vi "RT Main.vi"() -> ()   [LabVIEW 2021]
uses:
  Real-Time/Controls/Data FGV Action.ctl
  Program Files (x86)/National Instruments/LabVIEW 2021/ProjectTemplates/Source/myRIO/Oscilloscope/myRIO v1.1/Real-Time/Controls/Wave Parameters.ctl
  Program Files (x86)/National Instruments/LabVIEW 2021/ProjectTemplates/Source/myRIO/Oscilloscope/myRIO v1.1/Real-Time/Controls/Waveform Enum.ctl
  Program Files (x86)/National Instruments/LabVIEW 2021/ProjectTemplates/Source/myRIO/Oscilloscope/myRIO v1.1/Real-Time/Controls/Channel Selector.ctl
  <vilib>/Platform/TimedLoop/XDataNode/timing_clust.ctl
  <vilib>/Platform/TimedLoop/XDataNode/nitl_modes.ctl
  <vilib>/Platform/TimedLoop/XDataNode/wakeup.ctl
  Real-Time/Controls/Global Stop.vi
  <vilib>/FPGAPlugInAG/myRIO-1900/niLvFpga_Open_myRIO-1900.vi
  <vilib>/rvi/interface/common/dynamic/niFpgaDynamicAddResources.vi
  <vilib>/rvi/interface/common/niFpgaWaitOnOcc.vi
  <vilib>/Utility/error.llb/Error Cluster From Error Code.vi
  <vilib>/rvi/errors/niLvFpgaAdjustHostInterfaceError.vi
  <vilib>/myRIO/Common/Instrument Driver Framework/Utilities/vis/FPGA Ref Manager.vi
  <vilib>/myRIO/Common/Instrument Driver Framework/Utilities/vis/Ref Counter.vi
  <vilib>/FPGAPlugInAG/Dynamic/niLvFpga_Run_Dynamic.vi
  <vilib>/rvi/Analysis/host/Private/Sample Rate To Loop Time (ticks).vi
  <vilib>/FPGAPlugInAG/Dynamic/niLvFpga_Abort_Dynamic.vi
  <vilib>/FPGAPlugInAG/Dynamic/niLvFpga_Close_Dynamic.vi
  <vilib>/rvi/interface/nirviOpenFPGA/nirviOpenFPGA.xnode
  FPGA Bitfiles/ScopeBitFile2CH.lvbitx
  <vilib>/rvi/interface/nirviMethod/nirviMethod.xnode
  <vilib>/rvi/interface/nirviReadWriteControl/nirviReadWriteControl.xnode
  <vilib>/Platform/TimedLoop/XDataNode/XDataNode.xnode
  <vilib>/rvi/interface/nirviCloseFPGA/nirviCloseFPGA.xnode
  <vilib>/rvi/errors/niLvFpgaMergeErrorWithErrorCode.vi
  <vilib>/rvi/interface/Simulation/niFpgaSimulationCallBeginRW.vi
  <vilib>/myRIO/Instrument Drivers/Utilities/Utilities.lvlib
  <vilib>/Platform/TimedLoop/XDataNode/XDNodeRunTimeDep.lvlib
  <vilib>/rvi/Analysis/host/Public/NI_FpgaMspHost.lvlib
  <vilib>/FPGAPlugInAG/Dynamic/niLvFpga_ConfigureFifo_Dynamic.vi
  <vilib>/FPGAPlugInAG/Dynamic/niLvFpga_StartFifo_Dynamic.vi
  NiFpgaLv.dll
  <vilib>/FPGAPlugInAG/Dynamic/niLvFpga_ReadFifo_Dynamic.vi
panel:
  in  "Number of Elements":u32=1000
  out "Elements Remaining":u32
  out "error out":errorcluster
  in  "Stop":bool
  out "End?":bool
  # "Instructions\n1. Run RT Main.vi\n2. Open Desktop Main.vi\n3. Specify myRIO IP Address\n4. Run Desktop Main.vi"
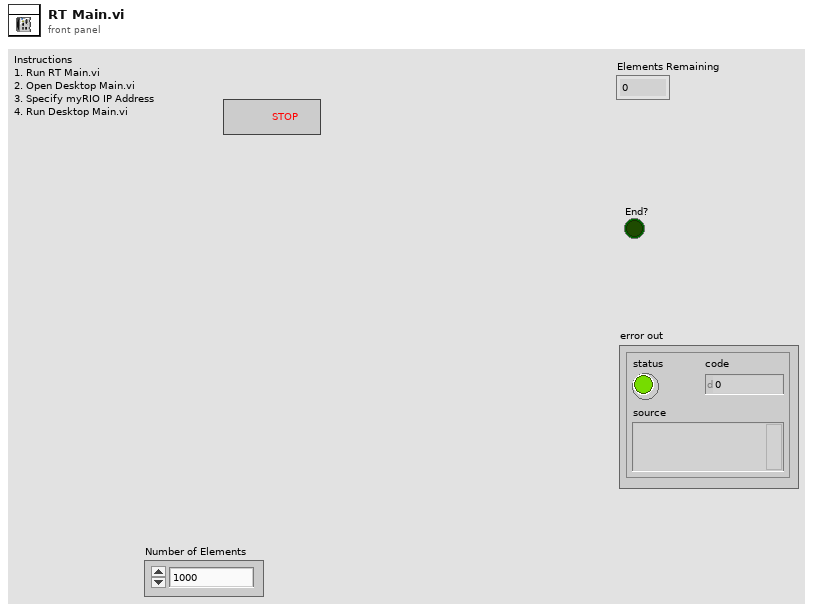
[diagram p1: front panel]
types:
  T1 = typedef "Data FGV Action.ctl" = enum16{"Initialize", "Set Scope Data", "Read Scope Data", "Set FGen", "Read FGen", "Set Params"}
  T2 = cluster{"read mode":enum16{"polling", "blocking"}, "write mode":enum16{"polling", "blocking"}}
  T3 = typedef "Wave Parameters.ctl" = cluster{"Frequency (Hz)":dbl, "Phase offset (deg)":dbl, "Vpeak (V)":dbl, "Offset (V)":dbl, "Waveform":T4, "Channel":T5}
  T4 = typedef "Waveform Enum.ctl" = enum16{"Sine", "Square"}
  T5 = typedef "Channel Selector.ctl" = enum16{"CH0", "CH1"}
  T6 = typedef "XDNodeRunTimeDep.lvlib/timing_clust.ctl" = cluster{"Expected End [f-1]":u64, "Actual End [f-1]":u64, "Finished Late? [f-1]":bool, "Expected End [i-1]":u64, "Actual End [i-1]":u64, "Finished Late? [i-1]":bool, "Expected Start [i]":u64, "Actual Start [i]":u64, "Expected Start [f]":u64, "Actual Start [f]":u64, "Source Name":string, "Structure Name":string, "Period":i64, "Deadline":i64, "Offset":i64, "Start":i64, "Priority":i32, "Timeout":i32, "Mode":T7, "Wakeup Reason":T8, "Error":errorcluster, "Source Type":string, "Secondary Source Type":string, "Global End Time":u64, "Global Start Time":u64, "Frame Duration":u64, "Iteration Duration":u64, "Assigned CPU":i32, "I/O Scan Engine Mode":u32}
  T7 = typedef "XDNodeRunTimeDep.lvlib/nitl_modes.ctl" = enum32{"No Change", "Process missed periods, maintain original phase", "Discard missed periods, maintain original phase", "Process missed periods, ignore original phase", "Discard missed periods, ignore original phase"}
  T8 = typedef "XDNodeRunTimeDep.lvlib/wakeup.ctl" = enum32{"Normal", "Aborted", "Asynchronous wakeup", "Timing source error", "Timed loop error", "Timeout"}
  T9 = typedef "Time Selector.ctl" = cluster{"Time/Div":T10}
  T10 = typedef "Time Knob.ctl" = dbl
  T11 = cluster{"Frequency (Hz)":bool, "Phase offset (deg)":bool, "Vpeak (V)":bool, "Offset (V)":bool, "Waveform":bool, "Channel":bool}
  T12 = typedef "Wave Properties - FPGA.ctl" = cluster{"Frequency (periods/tick)":fxp<+,32,0>, "Phase offset (periods)":fxp<+,32,0>, "Scale factor":fxp<+/-,24,1>, "Amplitude offset":fxp<+/-,24,12>, "Waveform":T4, "Channel":T5}
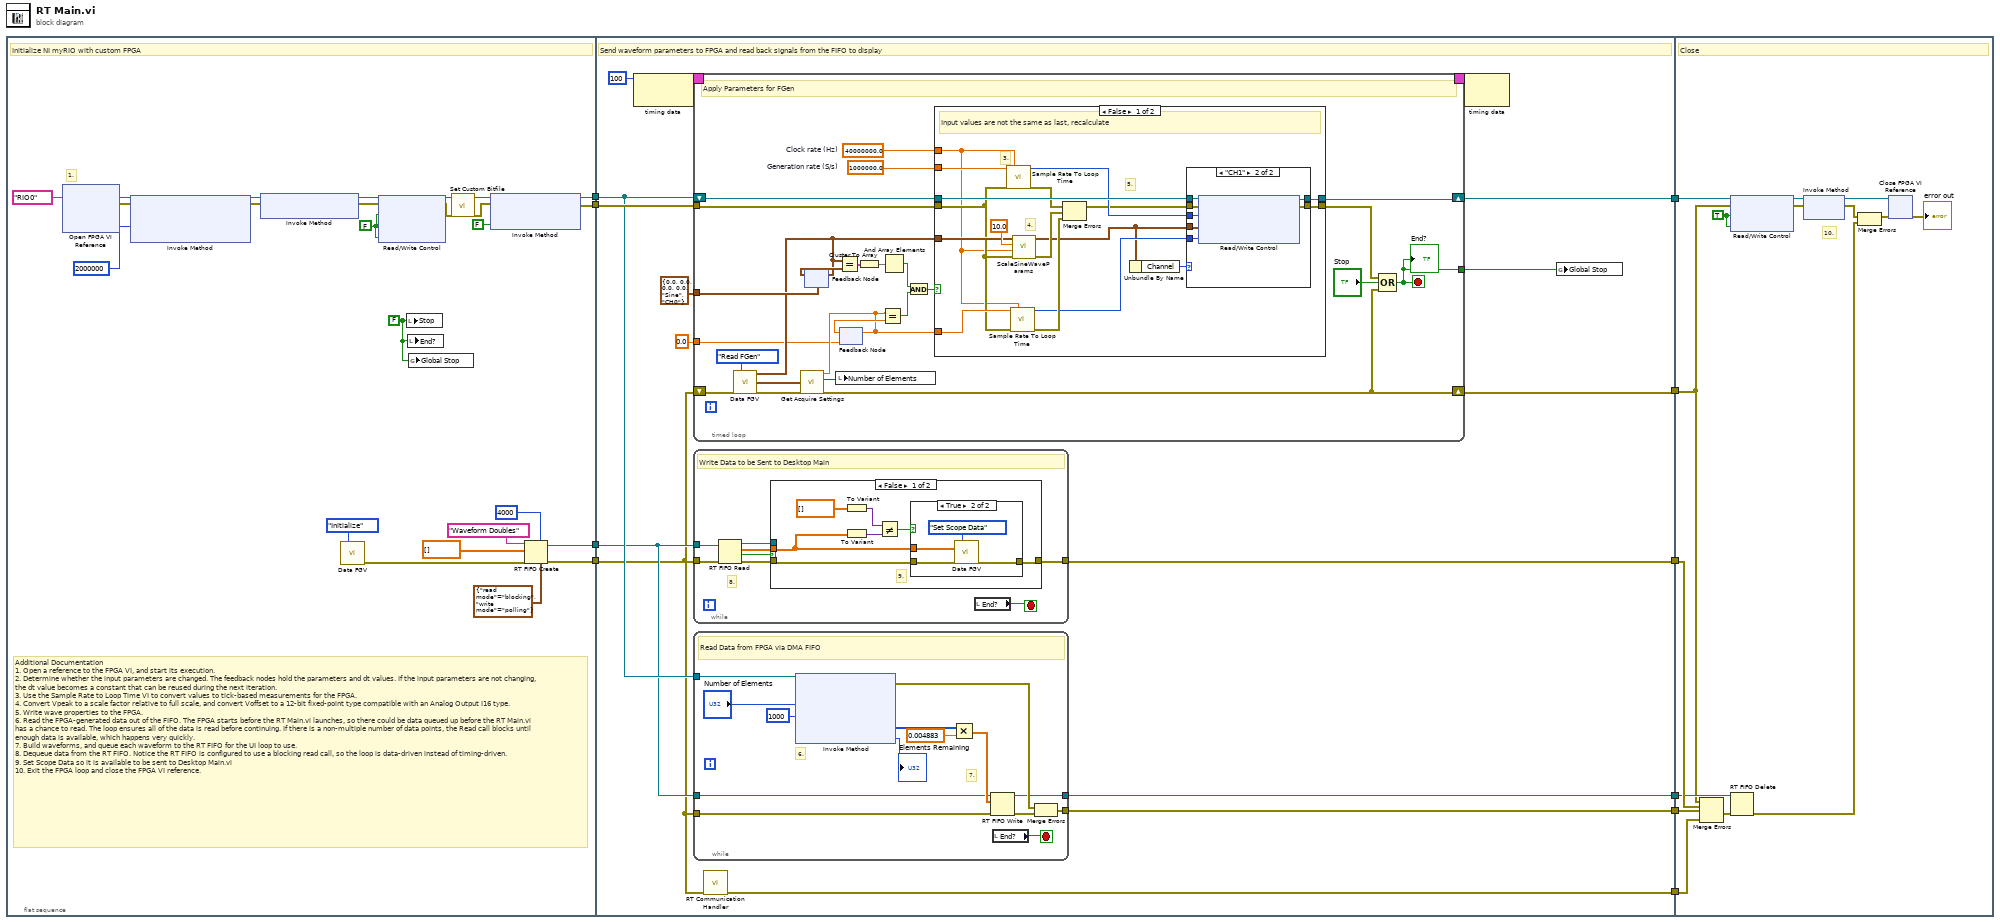
[diagram p0: block diagram]
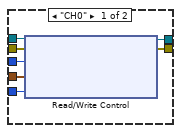
[diagram p4: hidden frame]
diagram:
  n1 = flat-sequence {
    tunnel: [w23] -> w10
    tunnel: [w22] -> w9
    tunnel: [w18] -> w6
    tunnel: [w17] -> w5
    tunnel: w10 -> [w44]
    tunnel: w9 -> [w51]
    tunnel: [w50] -> w8
    tunnel: [w45] -> w7
    tunnel: w6 -> [w37]
    tunnel: w5 -> [w42]
    tunnel: [w41] -> w4
    tunnel: [w40] -> w3
    tunnel: [w39] -> w2
    tunnel: [w36] -> w1
    tunnel: w8 -> [w165]
    tunnel: w7 -> [w151]
    tunnel: w4 -> [w158]
    tunnel: w3 -> [w157]
    tunnel: w2 -> [w156]
    tunnel: w1 -> [w152]
    frame #0 {
      w14 = FALSE ("Reset")
      w11 = FALSE ("Stop")
      # "Additional Documentation\n1. Open a reference to the FPGA VI, and start its execution.\n2. Determine whether the input parameters are changed. The feedback nodes hold the parameters and dt values. If the input parameters are not changing, the dt value becomes a constant that can be reused during the next iteration.\n3. Use the Sample Rate to Loop Time VI to convert values to tick-based measurements for the FPGA.\n4. Convert Vpeak to a scale factor relative to full scale, and convert Voffset to a 12-bit fixed-point type compatible with an Analog Output I16 type.\n5. Write wave properties to the FPGA. \n6. Read the FPGA-generated data out of the FIFO. The FPGA starts before the RT Main.vi launches, so there could be data queued up before the RT Main.vi has a chance to read. The loop ensures all of the data is read before continuing. If there is a non-multiple number of data points, the Read call blocks until enough data is available, which happens very quickly.\n7. Build waveforms, and queue each waveform to the RT FIFO for the UI loop to use.\n8. Dequeue data from the RT FIFO. Notice the RT FIFO is configured to use a blocking read call, so the loop is data-driven instead of timing-driven.\n9. Set Scope Data so it is available to be sent to Desktop Main.vi\n10. Exit the FPGA loop and close the FPGA VI reference."
      # "1."
      # "Initialize NI myRIO with custom FPGA"
      n2 = xnode "Open FPGA VI Reference"("resource name"=tag "RIO0") -> ("FPGA VI Reference Out"=w28:refnum<k20>, "error out"=w27:errorcluster)  [unwired: 1 in]
      n3 = xnode "Invoke Method"("FPGA VI Reference In"=w28, "error in"=w27, "Requested Depth"=u32 2000000) -> ("FPGA VI Reference Out"=w33:refnum<k20>, "error out"=w32:errorcluster)  [unwired: 1 out]
      n4 = xnode "Invoke Method"("FPGA VI Reference In"=w33, "error in"=w32) -> ("FPGA VI Reference Out"=w31:refnum<k20>, "error out"=w30:errorcluster)
      n5 = call "Data FGV.vi"("Action"=Data_FGV_Action."Initialize") -> ("error out"=w12:errorcluster)  [unwired: 10 in, 4 out]
      n6 = xnode "Read/Write Control"("FPGA VI Reference In"=w31, "error in"=w30, "Stop Output"=w11, "Initialize AO0"=w11, "Initialize AO1"=w11) -> ("FPGA VI Reference Out"=w29:refnum<k20>, "error out"=w26:errorcluster)
      n7 = local write "Stop"(w14) -> ()
      n8 = local write "End?"(w14) -> ()
      n9 = global write "Global Stop.vi" "Global Stop"(w14) -> ()
      n10 = call <vilib>:"Set Custom Bitfile.vi"("error in (no error)"=w26, "Custom FPGA Reference In"=w29) -> ("error out"=w24:errorcluster, "Custom FPGA Reference Out"=w25:refnum<k20>)  [unwired: 8 in]
      n11 = xnode "Invoke Method"("FPGA VI Reference In"=w25, "error in"=w24, "Wait Until Done (F)"=FALSE) -> ("FPGA VI Reference Out"=w23:refnum<k20>, "error out"=w22:errorcluster)
      n12 = RT FIFO Create(0:"Waveform Doubles" ("name (unnamed)"), 1:dbl[] [] ("x"), 3:w12, 6:u32 4000 ("size (10)"), 7:T2 {"read mode"=enum."blocking", "write mode"=enum."polling"} ("r/w modes (polling,polling)")) -> (8:w17:refnum<k33>, 11:w18:errorcluster)  [unwired: 3 in, 1 out]
    }
    frame #1 {
      # "Send waveform parameters to FPGA and read back signals from the FIFO to display"
      n13 = node-c288(i64 100 ("Period")) -> (w49:T6)
      n14 = while {
        tunnel: w42 -> [w72]
        tunnel: w37 -> [w67]
        tunnel: [w66] -> w40
        stop <- w73 stop-if-true
        # "8."
        # "Write Data to be Sent to Desktop Main"
        n15 = RT FIFO Read(0:w72, 3:w67) -> (8:w71:refnum<k33>, 9:w69:dbl[], 10:w68:bool, 11:w70:errorcluster)  [unwired: 2 in, 1 out]
        n16 = case shown="False" w68 {
          tunnel: w71 -> [_ _]
          tunnel: w70 -> [w75 w86]
          tunnel: w69 -> [w76 _]
          tunnel: [w74 w86] -> w66
          frame False {
            # "9."
            n17 = To Variant(anything=dbl[] [] ("x")) -> (Variant=w79:variant)
            n18 = To Variant(anything=w76) -> (Variant=w78:variant)
            n19 = Not Equal?(x=w79, y=w78) -> (x != y?=w77:bool)
            n20 = case shown="True" w77 {
              tunnel: w76 -> [_ w83]
              tunnel: w75 -> [w81 w85]
              tunnel: [w81 w82] -> w74
              frame False {
              }
              frame True {
                n21 = call "Data FGV.vi"("Action"=Data_FGV_Action."Set Scope Data", "Data"=w83, "error in (no error)"=w85) -> ("error out"=w82:errorcluster)  [unwired: 8 in, 4 out]
              }
            }
          }
          frame True {
          }
        }
        n22 = local read "End?"() -> (w73:bool)
      }
      n23 = timed-loop {
        shift-right: [w90] -> w50
        shift-left: w44 -> [w95]
        timing: w49 -> [_]
        timing-out: [_] -> w48
        shift-right: [w106] -> w45
        shift-left: w37 -> [w109]
        tunnel: T3 {"Frequency (Hz)"=0.0, "Phase offset (deg)"=0.0, "Vpeak (V)"=0.0, "Offset (V)"=0.0, "Waveform"=enum."Sine", "Channel"=enum."CH0"} ("Sinewave Props") -> [w92]
        tunnel: w51 -> [w94]
        tunnel: 0.0 ("Acq Rate(us)") -> [w87]
        tunnel: [w110] -> w38
        stop <- w110 stop-if-true
        w96 = 1000000.0  # Generation rate (S/s)
        w97 = 40000000.0  # Clock rate (Hz)
        # "Apply Parameters for FGen"
        n24 = call "Data FGV.vi"("Action"=Data_FGV_Action."Read FGen", "error in (no error)"=w109) -> ("Wave Parameters"=w91:T3, "Time"=w93:T9, "error out"=w107:errorcluster)  [unwired: 9 in, 2 out]
        n25 = call "Get Acquire Settings.vi"("error in (no error)"=w107, "Time"=w93) -> ("error out"=w106:errorcluster, "# Elements to Read"=w105:u32, "Acquire Rate"=w88:dbl)  [unwired: 7 in]
        n26 = feedback #1(w92) -> (w100:T3)
        n27 = feedback-in #1(w91) -> ()
        n28 = local write "Number of Elements"(w105) -> ()
        n29 = Equal?(x=w91, y=w100) -> (x = y?=w98:T11)
        n30 = feedback #2(w87) -> (w101:dbl)
        n31 = feedback-in #2(w88) -> ()
        n32 = Cluster To Array(cluster=w98) -> (array=w99:bool[])
        n33 = Equal?(x=w88, y=w101) -> (x = y?=w102:bool)
        n34 = And Array Elements(Boolean array=w99) -> (logical AND=w103:bool)
        n35 = And(x=w103, y=w102) -> (x .and. y?=w104:bool)
        n36 = case shown="False" w104 {
          tunnel: w95 -> [w128 w144]
          tunnel: w96 -> [w126 _]
          tunnel: w94 -> [w117 w143]
          tunnel: w91 -> [w119 _]
          tunnel: [w121 w144] -> w90
          tunnel: [w120 w143] -> w89
          tunnel: w97 -> [w114 _]
          tunnel: w88 -> [w118 _]
          frame False {
            # "3."
            # "5."
            # "4."
            # "Input values are not the same as last, recalculate"
            n37 = call-poly <vilib>:"Sample Rate To Loop Time.vi"("sample rate (S/s)"=w126, "FPGA clock rate (Hz)"=w114, "error in (no error)"=w117) -> ("count (ticks/S)"=w127:u32, "error out"=w123:errorcluster)  [unwired: 10 in, 1 out]
            n38 = call-poly <vilib>:"Sample Rate To Loop Time.vi"("sample rate (S/s)"=w118, "FPGA clock rate (Hz)"=w114, "error in (no error)"=w117) -> ("count (ticks/S)"=w115:u32, "error out"=w116:errorcluster)  [unwired: 10 in, 1 out]
            n39 = call "ScaleSineWaveParams.vi"("error in (no error)"=w117, "FPGA Clock Rate"=w114, "max voltage for target"=10.0, "Sine wave"=w119) -> ("error out"=w125:errorcluster, "Wave Props"=w113:T12)  [unwired: 6 in]
            n40 = Merge Errors(w123, w125, w116) -> (w124:errorcluster)
            n41 = Unbundle By Name(w113) -> ("Channel"=w112:T5)
            n42 = case shown="\"CH1\"" w112 {
              tunnel: w128 -> [w135 w142]
              tunnel: w127 -> [w134 w141]
              tunnel: w124 -> [w133 w140]
              tunnel: [w132 w139] -> w121
              tunnel: [w131 w138] -> w120
              tunnel: w115 -> [w130 w137]
              tunnel: w113 -> [w129 w136]
              frame "CH0" {
                n43 = xnode "Read/Write Control"("FPGA VI Reference In"=w135, "error in"=w133, "AO0 Loop Rate (ticks)"=w134, "Wave Properties AO0"=w129, "Acq Rate(ticks)"=w130) -> ("FPGA VI Reference Out"=w132:refnum<k20>, "error out"=w131:errorcluster)
              }
              frame "CH1" {
                n44 = xnode "Read/Write Control"("FPGA VI Reference In"=w142, "error in"=w140, "AO1 Loop Rate (ticks)"=w141, "Wave Properties AO1"=w136, "Acq Rate(ticks)"=w137) -> ("FPGA VI Reference Out"=w139:refnum<k20>, "error out"=w138:errorcluster)
              }
            }
          }
          frame True {
            # "Input values did not change, use previous values"
          }
        }
        n45 = Compound Arithmetic op=OR(w89, "Stop", w106) -> (w110:bool)
        "End?" <- w110
      }
      n46 = while {
        tunnel: w44 -> [w63]
        tunnel: w42 -> [w57]
        tunnel: w37 -> [w56]
        tunnel: [w53] -> w39
        tunnel: [w52] -> w41
        stop <- w60 stop-if-true
        # "7."
        # "6."
        # "Read Data from FPGA via DMA FIFO"
        n47 = xnode "Invoke Method"("FPGA VI Reference In"=w63, "Number of Elements"="Number of Elements", "Timeout (ms)"=1000) -> ("error out"=w54:errorcluster, "Data"=w59:i16[], "Elements Remaining"=→"Elements Remaining":u32)  [unwired: 1 in, 1 out]
        n48 = Multiply(x=w59, y=0.004883) -> (x*y=w58:dbl[])
        n49 = RT FIFO Write(0:w57, 1:w58, 3:w56) -> (8:w53:refnum<k33>, 11:w55:errorcluster)  [unwired: 2 in, 2 out]
        n50 = local read "End?"() -> (w60:bool)
        n51 = Merge Errors(w54, w55) -> (w52:errorcluster)
      }
      n52 = call "RT Communication Handler.vi"("error in (no error)"=w37) -> ("error out"=w36:errorcluster)  [unwired: 10 in]
      n53 = node-c288(w48) -> ()  [unwired: 1 out]
      n54 = global write "Global Stop.vi" "Global Stop"(w38) -> ()
    }
    frame #2 {
      w160 = TRUE ("Stop")
      # "10."
      # "Close"
      n55 = Merge Errors(w151, w157, w158, w152) -> (w159:errorcluster)
      n56 = xnode "Read/Write Control"("FPGA VI Reference In"=w165, "error in"=w151, "Stop Output"=w160, "Stop Input"=w160) -> ("FPGA VI Reference Out"=w164:refnum<k20>, "error out"=w163:errorcluster)
      n57 = RT FIFO Delete(0:w156, 3:w159) -> (11:w161:errorcluster)  [unwired: 1 in]
      n58 = xnode "Invoke Method"("FPGA VI Reference In"=w164, "error in"=w163) -> ("FPGA VI Reference Out"=w162:refnum<k20>, "error out"=w155:errorcluster)
      n59 = Merge Errors(w155, w161) -> (w154:errorcluster)
      n60 = xnode "Close FPGA VI Reference"("FPGA VI Reference In"=w162, "error in"=w154) -> ("error out"=→"error out":errorcluster)
    }
  }
